vi "initialize.vi"(0 "NInstrSim":refnum<class "NInstrSim.lvclass">, 3 "initializationData":variant, 5 "error in (no error)":errorcluster, 7 "binaryString":string, 8 "I8 Array":i8[](array[numeric]), 9 "prependSize? (T)":bool, 11 "byteOrder (0:big-endian, network order)":T1(ring)) -> (14 "dup NInstrSim":refnum<class "NInstrSim.lvclass">, 17 "found?":bool, 19 "error out":errorcluster)   [LabVIEW 2009, in "HB_Device_Examples.lvlib" / "NInstrSim.lvclass"]
doc: "This is a dynamic dispatch VI to be implemented by child classes to initialize their attributes.\n\n<B>Recommendation:</B> Use Variant for initialization data."
uses:
  NInstrSim.lvclass
  lib.lib/HGF_LVC/HGF_BaseClasses/HGF_TriggeredEvent/HGF_TriggeredEvent.lvclass
  lib.lib/HGF_LVC/HGF_DeviceBaseClasses/HGF_VISADevice/HGF_VISADevice.lvclass
  NInstrSim.lvclass/NInstrSim.ctl
  non_GPL/instr.lib/NI Instrument Simulator/NI Instrument Simulator.lvlib
  lib.lib/HGF_LVC/HGF_DeviceBaseClasses/HGF_DeviceBase/HGF_DeviceBase.lvclass
  lib.lib/HGF_LVC/HGF_BaseClasses/HGF_Factory/HGF_Factory.lvclass
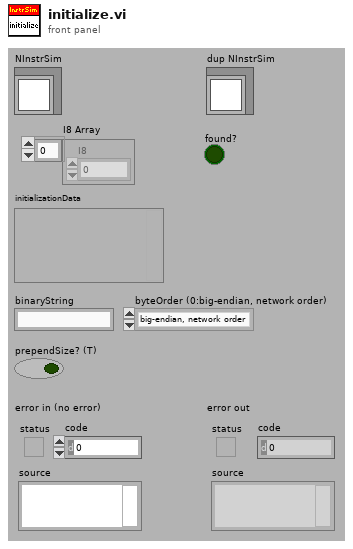
[diagram p1: front panel]
types:
  T1 = enum16{"big-endian, network order", "native, host order", "little-endian"}
  T2 = cluster{"Baud Rate":u32, "Flow Control":u16, "Parity":u16, "Data Bits":u16, "Stop Bits":u16}
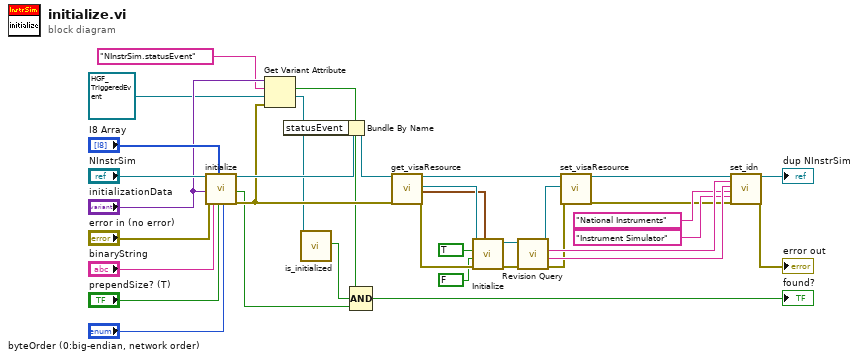
[diagram p0: block diagram]
diagram:
  n1 = call-parent "initialize.vi"("HGF_VISADevice"="NInstrSim", "initializationData"="initializationData", "error in (no error)"="error in (no error)", "binaryString"="binaryString", "I8 Array"="I8 Array", "prependSize? (T)"="prependSize? (T)", "byteOrder (0:big-endian, network order)"="byteOrder (0:big-endian, network order)") -> ("dup HGF_VISADevice"=w9:refnum<class "NInstrSim.lvclass">, "found?"=w5:bool, "error out"=w7:errorcluster)  [unwired: 10 out]
  n2 = Get Variant Attribute(Variant="initializationData", name="NInstrSim.statusEvent", default value (empty Variant)=refnum<class "HGF_TriggeredEvent.lvclass"> refnum ("Status_Event"), error in=w7) -> (found=w6:bool, value=w3:refnum<class "HGF_TriggeredEvent.lvclass">)  [unwired: 2 out]
  n3 = Bundle By Name(cluster=w9, "statusEvent"=w3) -> (w8:refnum<class "NInstrSim.lvclass">)
  n4 = call "is_initialized.vi"("HGF_Factory"=w3) -> ("initialized?"=w2:bool)  [unwired: 1 in, 17 out]
  n5 = Compound Arithmetic op=AND(w6, w2, w5) -> (→"found?":bool)
  n6 = call "get_visaResource.vi"("HGF_VISADevice"=w8, "error in (no error)"=w7) -> ("dup HGF_VISADevice"=w17:refnum<class "NInstrSim.lvclass">, "VISA Resource Name"=w28:refnum<visa-resource-name>, "Serial Configuration"=w12:T2, "error out"=w29:errorcluster)  [unwired: 14 out]
  n7 = call "Initialize.vi"("Serial Configuration"=w12, "error in (no error)"=w29, "Reset? (T: Yes)"=FALSE, "ID Query? (T: Yes)"=TRUE, "VISA resource name"=w28) -> ("error out"=w24:errorcluster, "VISA resource name out"=w25:refnum<visa-resource-name>)  [unwired: 5 out]
  n8 = call "Revision Query.vi"("error in (no error)"=w24, "VISA resource name"=w25) -> ("error out"=w15:errorcluster, "Instrument Firmware Revision"=w20:string, "Instrument Driver Revision"=w21:string, "VISA resource name out"=w13:refnum<visa-resource-name>)  [unwired: 6 out]
  n9 = call "set_visaResource.vi"("HGF_VISADevice"=w17, "visaResource"=w13, "error in (no error)"=w15) -> ("dup HGF_VISADevice"=w16:refnum<class "NInstrSim.lvclass">, "error out"=w14:errorcluster)  [unwired: 15 out]
  n10 = call "set_idn.vi"("HGF_DeviceBase"=w16, "driverRevision"=w21, "firmwareRevision"=w20, "vendor"="National Instruments", "model"="Instrument Simulator", "error in (no error)"=w14) -> ("dup HGF_DeviceBase"=→"dup NInstrSim":refnum<class "NInstrSim.lvclass">, "error out"=→"error out":errorcluster)  [unwired: 12 out]
